vi "Set Node Text Content.vi"(8 "error in (no error)":errorcluster, 10 "newValue":string, 11 "node in":refnum<k20>) -> (0 "error out":errorcluster, 2 "previousValue":string, 3 "node out":refnum<k20>)   [LabVIEW 2012]
doc: "SciScan 1.2 160622\nReturns the combined values of <B>Text_Node</B> children that the <B>node in</B> node owns."
uses:
  <vilib>/xml/Close Reference(Node).vi
  <vilib>/xml/NI_XML.lvlib
  <resource>/objmgr/DOMUserDefRef.rc
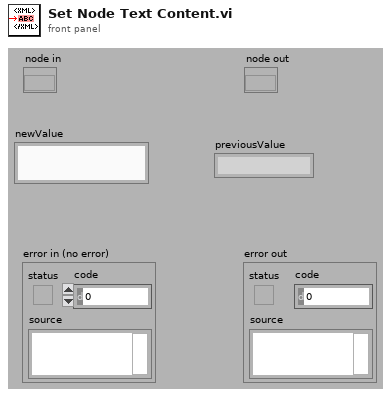
[diagram p1: front panel]
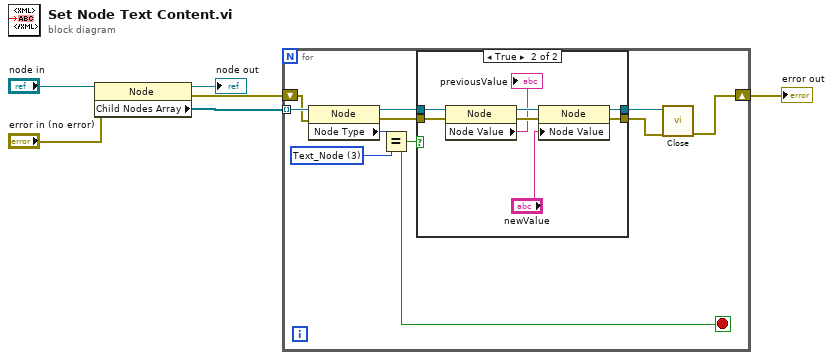
[diagram p0: block diagram]
diagram:
  n1 = property class="Node"(reference="node in", error in="error in (no error)") -> (reference out=→"node out":refnum<k20>, error out=w4:errorcluster, "Child Nodes Array"=w3:refnum<k20>[])
  n2 = for {
    shift-right: [w8] -> w1
    shift-left: w4 -> [w15]
    tunnel: w3 -> [w16] mode=indexing
    stop <- w7 stop-if-true
    w13 = 3 items=["Element_Node"=1, "Attribute_Node"=2, "Text_Node"=3, "CDATASection_Node"=4, "EntityReference_Node"=5, "Entity_Node"=6, "ProcessingInstruction_Node"=7, "Comment_Node"=8, "Document_Node"=9, "DocumentType_Node"=10, "DocumentFragment_Node"=11, "Notation_Node"=12] ("Node Type")
    n3 = property class="Node"(reference=w16, error in=w15) -> (reference out=w12:refnum<k20>, error out=w11:errorcluster, "Node Type"=w14:i32)
    n4 = Equal?(x=w14, y=w13) -> (x = y?=w7:bool)
    n5 = case shown="True" w7 {
      tunnel: w12 -> [w18 w23]
      tunnel: w11 -> [w17 w22]
      tunnel: [w18 w26] -> w10
      tunnel: [w17 w25] -> w9
      frame False {
      }
      frame True {
        n6 = property class="Node"(reference=w23, error in=w22) -> (reference out=w20:refnum<k20>, error out=w21:errorcluster, "Node Value"=→"previousValue":string)
        n7 = property class="Node"(reference=w20, error in=w21, "Node Value"="newValue") -> (reference out=w26:refnum<k20>, error out=w25:errorcluster)
      }
    }
    n8 = call-poly <vilib>:"Close.vi"("error in (no error)"=w9, "node"=w10) -> ("error out"=w8:errorcluster)  [unwired: 7 out]
  }
  "error out" <- w1
